vi "RunOxideCycle.vi"(10 "UiDefinition":T1) -> ()   [LabVIEW 2020]
uses:
  UIReferences.ctl
  C:/Users/User/Desktop/Automation/NextVersion4/LabviewDXFViewer/bin/Release/LabviewDXFViewer.exe
  LabviewDXFViewer/bin/Release/LabviewDXFViewer.exe
  <vilib>/Utility/file.llb/Write Delimited Spreadsheet (string).vi
  Keithley 2600 Series/Public/Configure/Source/Configure Source (Range).vi
  Keithley 2600 Series/Public/Configure/Source/Configure Source (Level).vi
  Keithley 2600 Series/Public/Configure/Source/Configure Source (Limit).vi
  Keithley 2600 Series/Public/Data/Read Measurement (Current).vi
  Keithley 2600 Series/Keithley 2600 Series.lvlib
panel:
  out "Current Buffer Data (A)":dbl[](array[numeric])
  out "Last Current (A)":dbl
  out "Leakage Current":dbl[][](array[numeric])
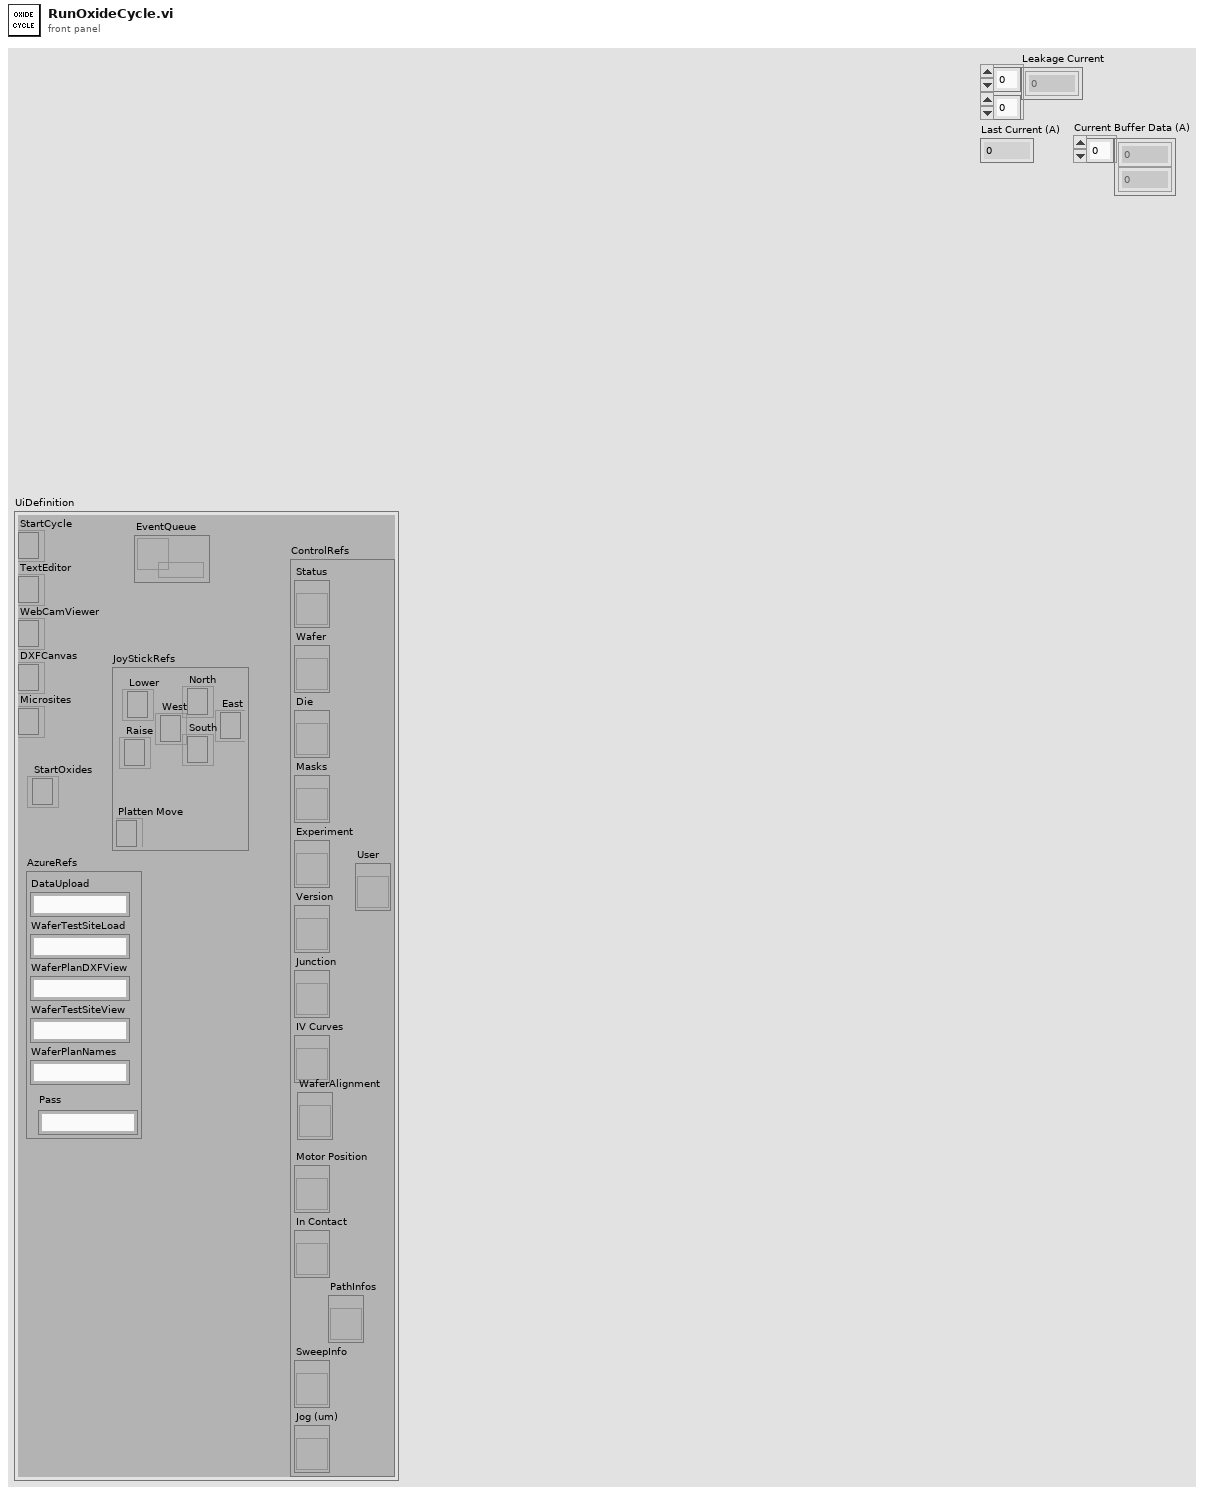
[diagram p1: front panel]
types:
  T1 = typedef "UIReferences.ctl" = cluster{"StartCycle":refnum<k24>, "TextEditor":refnum<k24>, "WebCamViewer":refnum<k24>, "DXFCanvas":refnum<k24>, "Microsites":refnum<k24>, "JoyStickRefs":cluster{"North":refnum<k24>, "Lower":refnum<k24>, "Raise":refnum<k24>, "Platten Move":refnum<k24>, "West":refnum<k24>, "East":refnum<k24>, "South":refnum<k24>}, "AzureRefs":cluster{"DataUpload":string, "WaferTestSiteLoad":string, "WaferPlanDXFView":string, "WaferTestSiteView":string, "WaferPlanNames":string, "Pass":string}, "ControlRefs":cluster{"Status":refnum<vi>, "Wafer":refnum<vi>, "Die":refnum<vi>, "Masks":refnum<vi>, "Experiment":refnum<vi>, "Version":refnum<vi>, "Junction":refnum<vi>, "IV Curves":refnum<vi>, "Motor Position":refnum<vi>, "In Contact":refnum<vi>, "SweepInfo":refnum<vi>, "Jog (um)":refnum<vi>, "PathInfos":refnum<vi>, "User":refnum<vi>, "WaferAlignment":refnum<vi>}, "EventQueue":refnum<queue>, "StartOxides":refnum<k24>}
  T2 = cluster{"Die":string, "Wafer":string, "Path":path, "url":string, "Experiment":string, "Version":string, "user":string}
  T3 = typedef "WaferAlignmentType.ctl" = cluster{"Wafer Units to microns":dbl, "Rotation Misalign":dbl[], "Scale Misalign":dbl, "Steps Per micron":dbl, "Position 1":i32[], "Chip Orientation":i32, "Position 2":i32[], "Lift Distance":i32, "Position 3":i32[], "Jog Height":i32}
  T4 = cluster{"Coordinates":dbl[], "Junction Name":string, "Orientation":string}[]
  T5 = cluster{"Current Range":dbl, "Source Measure Unit Channel (0: Channel A)":i32, "Waveform":waveform(dbl), "VISA resource name":refnum<visa-resource-name>, "CodeText":string}
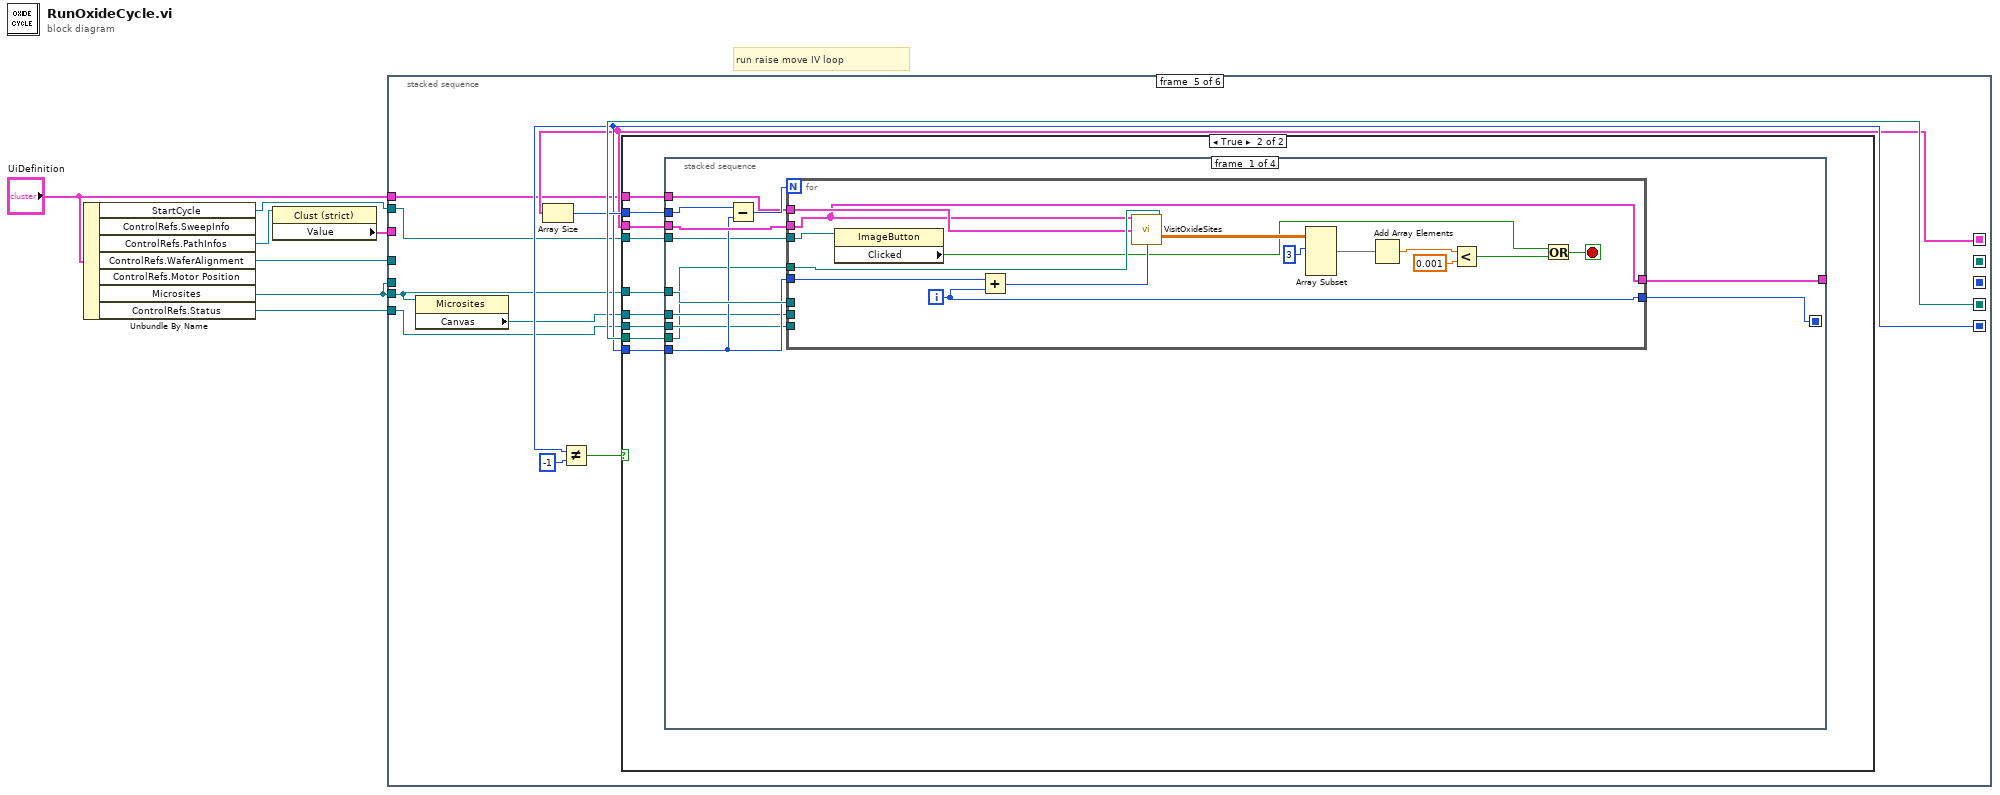
[diagram p0: block diagram]
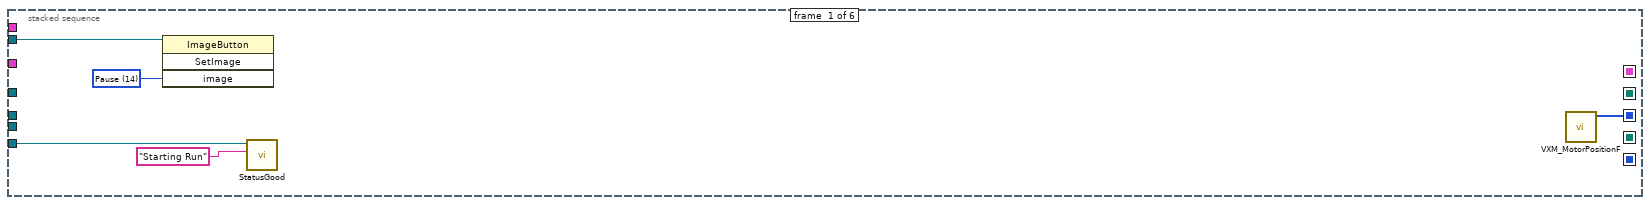
[diagram p2: hidden frame]
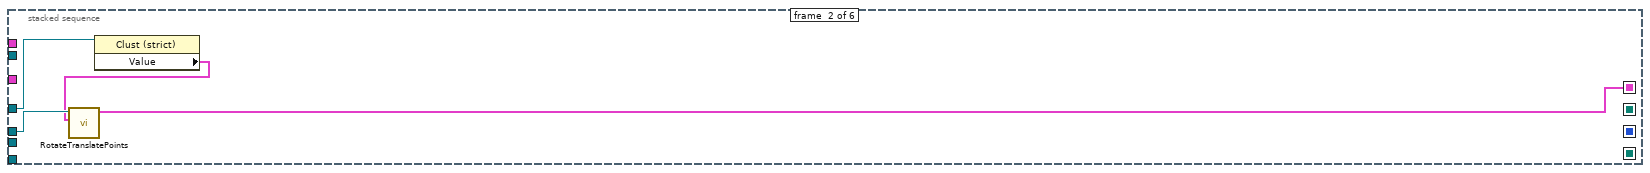
[diagram p3: hidden frame]
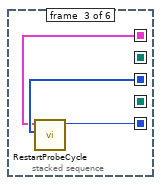
[diagram p4: hidden frame]
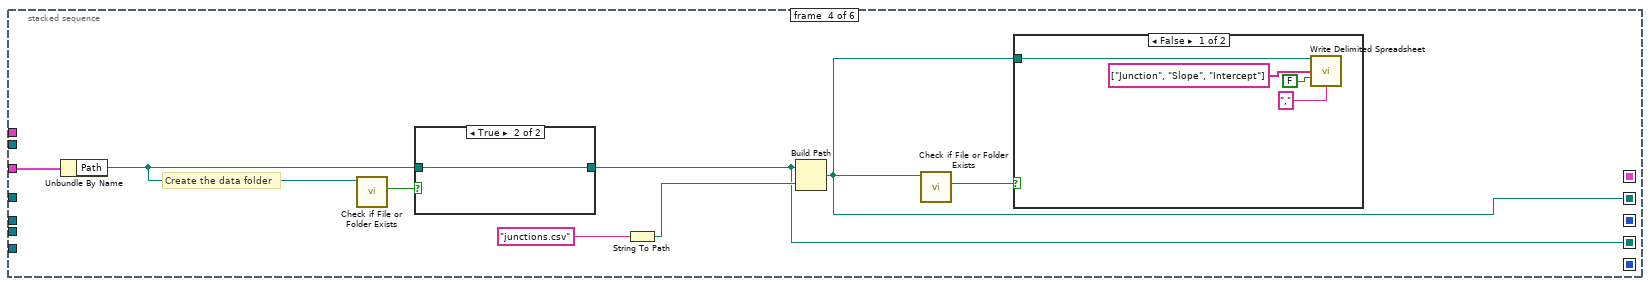
[diagram p5: hidden frame]
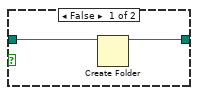
[diagram p7: hidden frame]
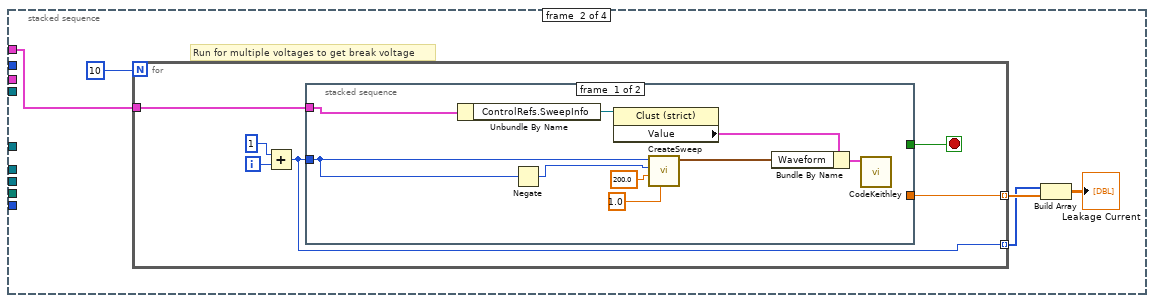
[diagram p9: hidden frame]
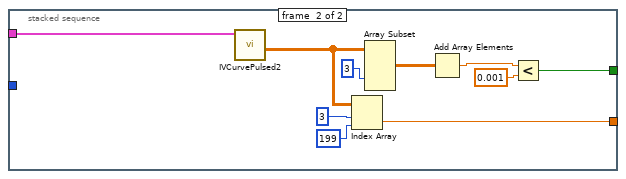
[diagram p10: hidden frame]
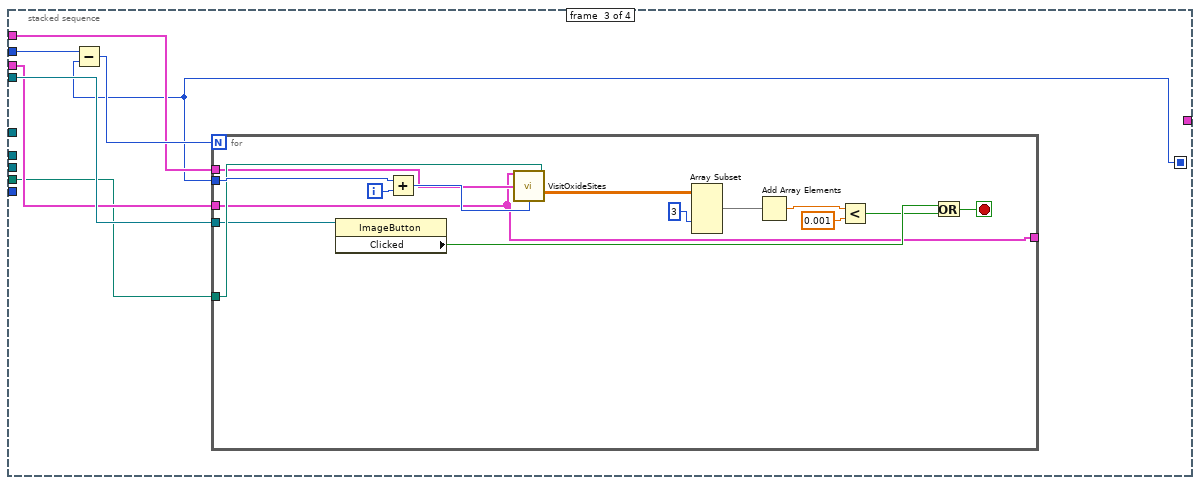
[diagram p11: hidden frame]
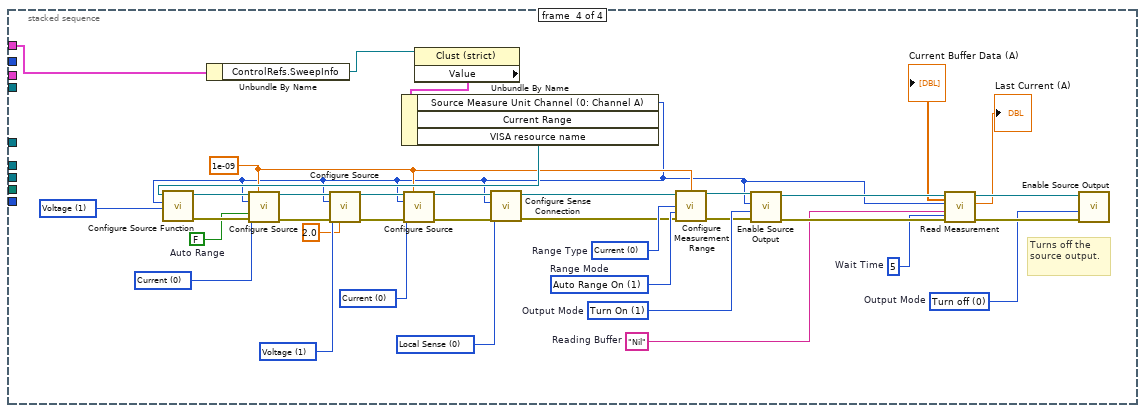
[diagram p12: hidden frame]
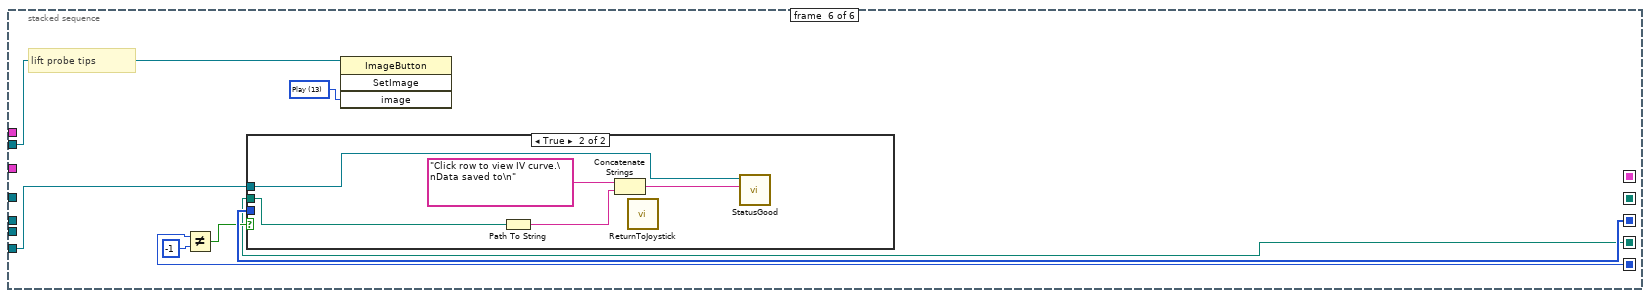
[diagram p13: hidden frame]
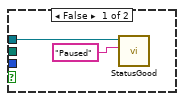
[diagram p14: hidden frame]
diagram:
  # "run raise move IV loop"
  n1 = Unbundle By Name("UiDefinition") -> ("StartCycle"=w7:refnum<k24>, "ControlRefs.PathInfos"=w5:refnum<vi>, "ControlRefs.WaferAlignment"=w1:refnum<vi>, "Microsites"=w3:refnum<k24>, "ControlRefs.Status"=w4:refnum<vi>)  [unwired: 2 out]
  n2 = property class="Clust (strict)"(reference=w5) -> ("Value"=w6:T2)  [unwired: 1 in, 2 out]
  n3 = stacked-sequence {
    seq-local: [_ w16 _ _ _ _] -> [_ _ w17 _ w36 _]
    seq-local: [w12 _ _ _ _ _] -> [_ _ w18 _ _ w178]
    seq-local: [_ _ _ w23 _ _] -> [_ _ _ _ w45 w172]
    seq-local: [_ _ w19 _ _ _] -> [_ _ _ _ w43 w176]
    seq-local: [_ _ _ w20 _ _] -> [_ _ _ _ _ _]
    tunnel: w3 -> [_ _ _ _ w37 _]
    tunnel: w6 -> [_ _ _ w24 _ _]
    tunnel: w7 -> [w11 _ _ _ w40 w174]
    tunnel: w4 -> [w8 _ _ _ w39 w171]
    tunnel: w3 -> [_ w15 _ _ _ _]
    tunnel: "UiDefinition" -> [_ _ _ _ w35 _]
    tunnel: w1 -> [_ w14 _ _ _ _]
    frame #0 {
      w10 = 14 items=["Left", "LeftBig", "LeftSmall", "Right", "RightBig", "RightSmall", "Up", "UpBig", "UpSmall", "Down", "DownBig", "DownSmall", "Zero", "Play", "Pause", "Load", "Lower", "Raise", "Home", "Home2"] ("image")
      n4 = invoke class="ImageButton" method="SetImage"(reference=w11, "image"=w10) -> ()  [unwired: 2 in, 4 out]
      n5 = call "StatusGood.vi"("Text.Text"="Starting Run" ("Run Message"), "String in"=w8) -> ()  [unwired: 10 in]
      n6 = call "VXM_MotorPositionF.vi"() -> ("Position"=w12:i32[])  [unwired: 11 in]
    }
    frame #1 {
      n7 = property class="Clust (strict)"(reference=w14) -> ("Value"=w13:T3)  [unwired: 1 in, 2 out]
      n8 = call "RotateTranslatePoints.vi"("WaferAlignment"=w13, ".NET Refnum in"=w15) -> ("Array"=w16:T4)  [unwired: 8 in, 1 out]
    }
    frame #2 {
      n9 = call "RestartProbeCycle.vi"("Position"=w18, "Array"=w17) -> ("Numeric"=w19:i32)  [unwired: 9 in]
    }
    frame #3 {
      # "Create the data folder"
      n10 = Unbundle By Name(w24) -> ("Path"=w22:path)
      n11 = call <vilib>:"Check if File or Folder Exists.vi"("path"=w22) -> ("file or folder exists?"=w27:bool)  [unwired: 8 in, 2 out]
      n12 = case shown="True" w27 {
        tunnel: w22 -> [w33 w34]
        tunnel: [w32 w34] -> w23
        frame False {
          n13 = Create Folder(path (use dialog)=w33) -> (created path=w32:path)  [unwired: 2 in, 2 out]
        }
        frame True {
        }
      }
      n14 = String To Path(string="junctions.csv") -> (path=w26:path)
      n15 = Build Path(base path=w23, name or relative path=w26) -> (appended path=w20:path)
      n16 = call <vilib>:"Check if File or Folder Exists.vi"("path"=w20) -> ("file or folder exists?"=w21:bool)  [unwired: 8 in, 2 out]
      n17 = case shown="False" w21 {
        tunnel: w20 -> [w31 _]
        frame False {
          n18 = call-poly <vilib>:"Write Delimited Spreadsheet.vi"("file path (dialog if empty)"=w31, "1D data"=string[] ["Junction", "Slope", "Intercept"], "append to file? (new file:F)"=FALSE, "delimiter (\\t)"="," ("delimiter (\\t)")) -> ()  [unwired: 10 in, 2 out]
        }
        frame True {
        }
      }
    }
    frame #4 {
      n19 = property class="Microsites"(reference=w37) -> ("Canvas"=w38:refnum<k24>)  [unwired: 1 in, 2 out]
      n20 = Array Size(array=w36) -> (size(s)=w44:i32)
      n21 = Not Equal?(x=w43, y=-1) -> (x != y?=w42:bool)
      n22 = case shown="True" w42 {
        tunnel: w36 -> [_ w54]
        tunnel: w37 -> [_ w53]
        tunnel: w45 -> [_ w48]
        tunnel: w43 -> [_ w52]
        tunnel: w44 -> [_ w49]
        tunnel: w40 -> [_ w47]
        tunnel: w39 -> [_ w51]
        tunnel: w38 -> [_ w50]
        tunnel: w35 -> [_ w46]
        frame False {
        }
        frame True {
          n23 = stacked-sequence {
            seq-local: [w55 _ _ _] -> [_ _ w112 _]
            tunnel: w54 -> [w66 _ w114 _]
            tunnel: w53 -> [w65 _ _ _]
            tunnel: w52 -> [w63 _ _ _]
            tunnel: w51 -> [w62 _ _ _]
            tunnel: w50 -> [w61 _ _ _]
            tunnel: w49 -> [w60 _ w115 _]
            tunnel: w48 -> [w59 _ w113 _]
            tunnel: [w56 _ _ _] -> _
            tunnel: w47 -> [w58 _ w117 _]
            tunnel: w46 -> [w57 w83 w116 w145]
            frame #0 {
              n24 = Subtract(x=w60, y=w63) -> (x-y=w64:i32)
              n25 = for {
                N: w64 -> [_]
                tunnel: w66 -> [w68]
                tunnel: w65 -> [_]
                tunnel: w59 -> [w80]
                tunnel: w63 -> [w81]
                tunnel: w58 -> [w77]
                tunnel: w62 -> [_]
                tunnel: w61 -> [_]
                tunnel: w57 -> [w78]
                tunnel: [w69] -> w55
                tunnel: [w68] -> w56
                i -> [w69]
                stop <- w70 stop-if-true
                n26 = property class="ImageButton"(reference=w77) -> ("Clicked"=w74:bool)  [unwired: 1 in, 2 out]
                n27 = Add(x=w81, y=w69) -> (x+y=w79:i32)
                n28 = call "VisitOxideSites.vi"("Microsites"=w68, "Path"=w80, "UiDefinition"=w78, "CurrentPositionIndex"=w79) -> ("IV"=w76:dbl[][])  [unwired: 11 in]
                n29 = Array Subset(array=w76, index (row)=3 ("index")) -> (w75:dbl[][])  [unwired: 3 in]
                n30 = Add Array Elements(numeric array=w75) -> (sum=w72:dbl)
                n31 = Less?(x=w72, y=0.001) -> (x < y?=w73:bool)
                n32 = Or(x=w74, y=w73) -> (x .or. y?=w70:bool)
              }
            }
            frame #1 {
              # "Run for multiple voltages to get break voltage"
              n33 = for {
                N: 10 -> [_]
                tunnel: w83 -> [w92]
                tunnel: [w88] -> w85 mode=indexing
                tunnel: [w87] -> w82 mode=indexing
                i -> [w91]
                stop <- w89 stop-if-true
                n34 = Add(x=1, y=w91) -> (x+y=w87:i32)
                n35 = stacked-sequence {
                  tunnel: w92 -> [w96 w103]
                  tunnel: w87 -> [w93 _]
                  tunnel: [_ w107] -> w89
                  tunnel: [_ w104] -> w88
                  frame #0 {
                    n36 = Unbundle By Name(w96) -> ("ControlRefs.SweepInfo"=w98:refnum<vi>)
                    n37 = Negate(x=w93) -> (-x=w94:i32)
                    n38 = property class="Clust (strict)"(reference=w98) -> ("Value"=w99:T5)  [unwired: 1 in, 2 out]
                    n39 = call "CreateSweep.vi"("Sweeps"=1.0, "Number Points"=200.0, "Minimum Voltage"=w94, "Maxiumum Voltage"=w93) -> ("Waveform"=w97:waveform(dbl))  [unwired: 6 in, 1 out]
                    n40 = Bundle By Name(cluster=w99, "Waveform"=w97) -> (w95:T5)
                    n41 = call "CodeKeithley.vi"("SweepInfo"=w95) -> ()  [unwired: 10 in, 1 out]
                  }
                  frame #1 {
                    n42 = call "IVCurvePulsed2.vi"("UiDefinition"=w103) -> ("appended array"=w102:dbl[][])  [unwired: 9 in, 1 out]
                    n43 = Index Array(array=w102, index (row)=3, index (col)=199 ("disabled index (col)")) -> (element=w104:dbl)
                    n44 = Array Subset(array=w102, index (col)=3 ("index")) -> (w110:dbl[][])  [unwired: 3 in]
                    n45 = Add Array Elements(numeric array=w110) -> (sum=w109:dbl)
                    n46 = Less?(x=w109, y=0.001) -> (x < y?=w107:bool)
                  }
                }
              }
              n47 = Build Array(w82, w85) -> (→"Leakage Current":dbl[][])
            }
            frame #2 {
              n48 = Subtract(x=w115, y=w112) -> (x-y=w118:i32)
              n49 = for {
                N: w118 -> [_]
                tunnel: w114 -> [w119]
                tunnel: w113 -> [w132]
                tunnel: w112 -> [w133]
                tunnel: w117 -> [w129]
                tunnel: w116 -> [w130]
                tunnel: [w119] -> _
                i -> [w120]
                stop <- w121 stop-if-true
                n50 = property class="ImageButton"(reference=w129) -> ("Clicked"=w125:bool)  [unwired: 1 in, 2 out]
                n51 = Add(x=w133, y=w120) -> (x+y=w131:i32)
                n52 = call "VisitOxideSites.vi"("Microsites"=w119, "Path"=w132, "UiDefinition"=w130, "CurrentPositionIndex"=w131) -> ("IV"=w128:dbl[][])  [unwired: 11 in]
                n53 = Array Subset(array=w128, index (col)=3 ("index")) -> (w126:dbl[][])  [unwired: 3 in]
                n54 = Add Array Elements(numeric array=w126) -> (sum=w123:dbl)
                n55 = Less?(x=w123, y=0.001) -> (x < y?=w124:bool)
                n56 = Or(x=w125, y=w124) -> (x .or. y?=w121:bool)
              }
            }
            frame #3 {
              w139 = 1 items=["Current", "Voltage"] ("Level Type (1: Voltage)")
              w146 = 0 items=["Current", "Voltage", "Power"] ("Limit Type (1: Voltage)")
              w153 = 0 items=["Local Sense", "Remote Sense"] ("Sense Mode (0: Local Sense)")
              w140 = 0 items=["Current", "Voltage"] ("Range Type (1: Voltage)")
              w137 = 1e-09 ("Current Range (1E-7 A)")
              w141 = 1 items=["Current", "Voltage"] ("Source Function (1: Voltage)")
              w151 = 1 items=["Auto Range Off", "Auto Range On", "Auto Range Follow Limit"]  # Range Mode
              w152 = 0 items=["Current", "Voltage"]  # Range Type
              w156 = 0 items=["Turn off", "Turn On", "High-Z"]  # Output Mode
              w159 = 5  # Wait Time
              w163 = 1 items=["Turn off", "Turn On", "High-Z"]  # Output Mode
              w160 = "Nil"  # Reading Buffer
              w166 = FALSE  # Auto Range
              # "Turns off the source output."
              n57 = Unbundle By Name(w145) -> ("ControlRefs.SweepInfo"=w144:refnum<vi>)
              n58 = property class="Clust (strict)"(reference=w144) -> ("Value"=w143:T5)  [unwired: 1 in, 2 out]
              n59 = Unbundle By Name(w143) -> ("Source Measure Unit Channel (0: Channel A)"=w136:i32, "VISA resource name"=w142:refnum<visa-resource-name>)  [unwired: 1 out]
              n60 = call "Configure Source Function.vi"("Source Function (1: Voltage)"=w141, "Source Measure Unit Channel (0: Channel A)"=w136, "VISA resource name"=w142) -> ("error out"=w169:errorcluster, "VISA resource name out"=w170:refnum<visa-resource-name>)  [unwired: 7 in]
              n61 = call-poly "Configure Source.vi"("VISA resource name"=w170, "Current Range (1E-7 A)"=w137, "Source Measure Unit Channel (0: Channel A)"=w136, "Range Type (1: Voltage)"=w140, "Auto Range (T: Enable)"=w166, "error in (no error)"=w169) -> ("VISA resource name out"=w168:refnum<visa-resource-name>, "error out"=w167:errorcluster)  [unwired: 8 in]
              n62 = call-poly "Configure Source.vi"("VISA resource name"=w168, "Source Measure Unit Channel (0: Channel A)"=w136, "Level Type (1: Voltage)"=w139, "error in (no error)"=w167, "Voltage Level (0 V)"=2.0) -> ("VISA resource name out"=w165:refnum<visa-resource-name>, "error out"=w164:errorcluster)  [unwired: 9 in]
              n63 = call-poly "Configure Source.vi"("VISA resource name"=w165, "Current Limit (0.1 A)"=w137, "Source Measure Unit Channel (0: Channel A)"=w136, "Limit Type (1: Voltage)"=w146, "error in (no error)"=w164) -> ("VISA resource name out"=w155:refnum<visa-resource-name>, "error out"=w154:errorcluster)  [unwired: 9 in]
              n64 = call "Configure Sense Connection.vi"("error in (no error)"=w154, "Sense Mode (0: Local Sense)"=w153, "Source Measure Unit Channel (0: Channel A)"=w136, "VISA resource name"=w155) -> ("error out"=w147:errorcluster, "VISA resource name out"=w148:refnum<visa-resource-name>)  [unwired: 6 in]
              n65 = call "Configure Measurement Range.vi"("VISA resource name"=w148, "Minimum Current Range (0.1 A)"=w137, "Range Type (0: Current)"=w152, "Range Mode (1: Auto Range On)"=w151, "error in (no error)"=w147) -> ("VISA resource name out"=w150:refnum<visa-resource-name>, "error out"=w149:errorcluster)  [unwired: 9 in]
              n66 = call "Enable Source Output.vi"("error in (no error)"=w149, "Output Mode (0: Turn off)"=w163, "Source Measure Unit Channel (0: Channel A)"=w136, "VISA resource name"=w150) -> ("error out"=w161:errorcluster, "VISA resource name out"=w162:refnum<visa-resource-name>)  [unwired: 6 in]
              n67 = call-poly "Read Measurement.vi"("Wait Time (10 S)"=w159, "error in (no error)"=w161, "Current Buffer (smua.nvbuffer1)"=w160, "Source Measure Unit Channel (0: Channel A)"=w136, "VISA resource name"=w162) -> ("error out"=w157:errorcluster, "Last Current (A)"=→"Last Current (A)":dbl, "VISA resource name out"=w158:refnum<visa-resource-name>, "Current Buffer Data (A)"=→"Current Buffer Data (A)":dbl[])  [unwired: 3 in]
              n68 = call "Enable Source Output.vi"("error in (no error)"=w157, "Output Mode (0: Turn off)"=w156, "VISA resource name"=w158) -> ()  [unwired: 7 in, 2 out]
            }
          }
        }
      }
    }
    frame #5 {
      w173 = 13 items=["Left", "LeftBig", "LeftSmall", "Right", "RightBig", "RightSmall", "Up", "UpBig", "UpSmall", "Down", "DownBig", "DownSmall", "Zero", "Play", "Pause", "Load", "Lower", "Raise", "Home", "Home2"] ("image")
      # "lift probe tips"
      n69 = Not Equal?(x=w176, y=-1) -> (x != y?=w175:bool)
      n70 = case shown="True" w175 {
        tunnel: w178 -> [_ _]
        tunnel: w172 -> [_ w185]
        tunnel: w171 -> [w180 w184]
        frame False {
          n71 = call "StatusGood.vi"("Text.Text"="Paused", "String in"=w180) -> ()  [unwired: 10 in]
        }
        frame True {
          n72 = Path To String(path=w185) -> (string=w183:string)
          n73 = Concatenate Strings("Click row to view IV curve.\nData saved to\n" ("Text.Text"), w183) -> (w181:string)
          n74 = call "ReturnToJoystick.vi"() -> ()  [unwired: 12 in]
          n75 = call "StatusGood.vi"("Text.Text"=w181, "String in"=w184) -> ()  [unwired: 10 in]
        }
      }
      n76 = invoke class="ImageButton" method="SetImage"(reference=w174, "image"=w173) -> ()  [unwired: 2 in, 4 out]
    }
  }
